vi "Save_File.vi"(6 "Sequence caption in":string, 7 "Path?":bool, 8 "error in (no error)":errorcluster, 9 "Sequence in":string[](array[string]), 10 "Buffer in":string[](array[string]), 11 "Path in":path) -> (0 "error out":errorcluster, 1 "Sequence out":string[](array[string]), 2 "Buffer out":string[](array[string]), 3 "Path out":path, 4 "Sequence caption out":string)   [LabVIEW 2025]
uses:
  <vilib>/Utility/file.llb/Write Delimited Spreadsheet (string).vi
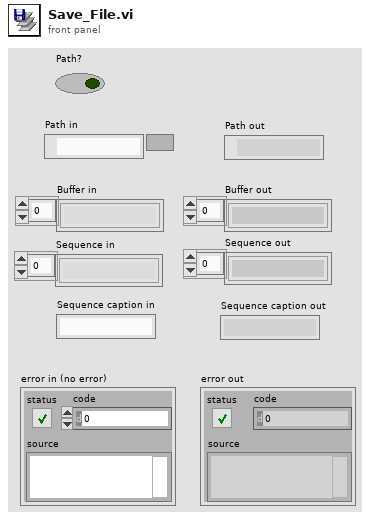
[diagram p1: front panel]
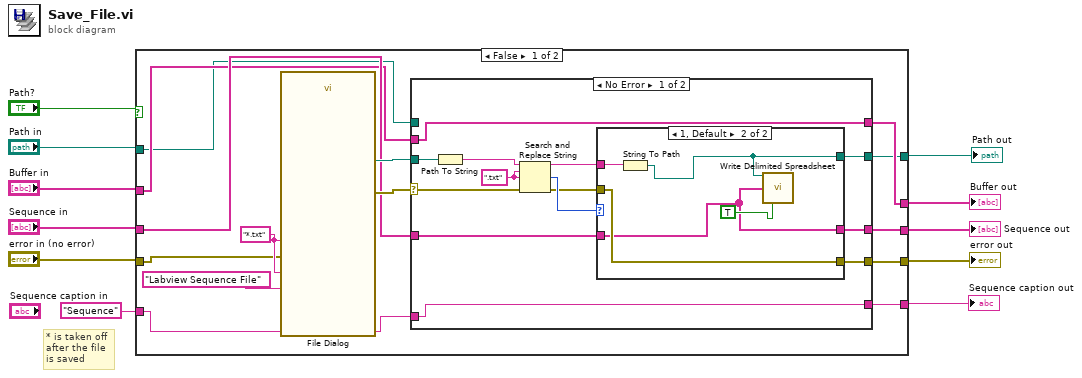
[diagram p0: block diagram]
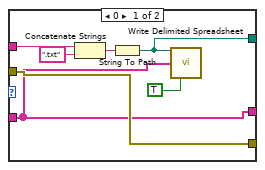
[diagram p2: hidden frame]
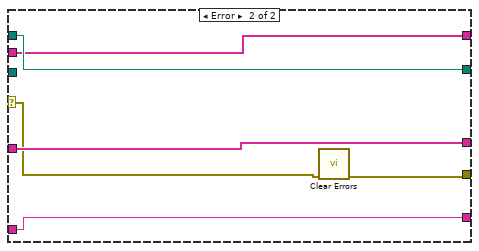
[diagram p3: hidden frame]
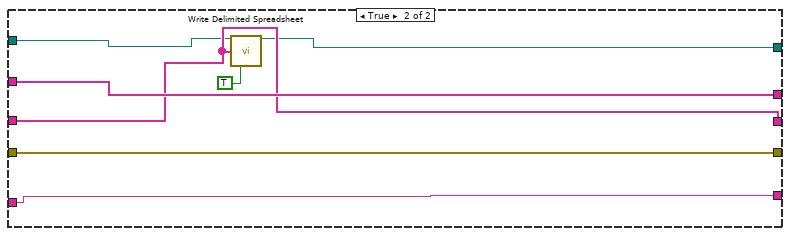
[diagram p4: hidden frame]
diagram:
  # "* is taken off\nafter the file\nis saved"
  n1 = case shown="False" "Path?" {
    tunnel: "Path in" -> [w12 w59]
    tunnel: "Buffer in" -> [w15 w63]
    tunnel: "Sequence in" -> [w18 w60]
    tunnel: "error in (no error)" -> [w21 w62]
    tunnel: [w13 w58] -> w6
    tunnel: [w14 w63] -> w5
    tunnel: [w17 w62] -> w3
    tunnel: [w16 w60] -> w4
    tunnel: "Sequence" ("Sequence caption in") -> [w20 w61]
    tunnel: [w19 w61] -> w2
    frame False {
      w25 = "*.txt" ("default name")
      n2 = call "File Dialog"("default name"=w25, "error in"=w21, "pattern (all files)"=w25, "pattern label"="Labview Sequence File") -> ("selected path"=w23:path, "error out"=w24:errorcluster)  [unwired: 8 in, 2 out]
      n3 = case shown="No Error" w24 {
        selector: w24 -> [w35 w52]
        tunnel: w23 -> [w36 _]
        tunnel: w20 -> [w29 w56]
        tunnel: [w29 w56] -> w19
        tunnel: w18 -> [w32 w55]
        tunnel: [w30 w51] -> w17
        tunnel: [w28 w55] -> w16
        tunnel: w15 -> [w27 w53]
        tunnel: [w27 w53] -> w14
        tunnel: [w26 w54] -> w13
        tunnel: w12 -> [_ w54]
        frame No Error {
          w37 = ".txt" ("search string")
          n4 = Path To String(path=w36) -> (string=w38:string)
          n5 = Search and Replace String(input string=w38, search string=w37, replace string=w37, error in=w35) -> (result string=w33:string, number of replacements=w34:i32, error out=w31:errorcluster)  [unwired: 4 in, 1 out]
          n6 = case shown="1, Default" w34 {
            tunnel: w33 -> [w45 w50]
            tunnel: w32 -> [w40 w46]
            tunnel: w31 -> [w42 w49]
            tunnel: [w42 w49] -> w30
            tunnel: [w40 w46] -> w28
            tunnel: [w39 w48] -> w26
            frame 0 {
              n7 = Concatenate Strings(w45, ".txt" ("string")) -> (w43:string)
              n8 = String To Path(string=w43) -> (path=w39:path)
              n9 = call-poly <vilib>:"Write Delimited Spreadsheet.vi"("file path (dialog if empty)"=w39, "1D data"=w40, "transpose? (no:F)"=TRUE) -> ()  [unwired: 11 in, 2 out]
            }
            frame 1, Default {
              n10 = String To Path(string=w50) -> (path=w48:path)
              n11 = call-poly <vilib>:"Write Delimited Spreadsheet.vi"("file path (dialog if empty)"=w48, "1D data"=w46, "transpose? (no:F)"=TRUE) -> ()  [unwired: 11 in, 2 out]
            }
          }
        }
        frame Error {
          n12 = call <vilib>:"Clear Errors.vi"("error in (no error)"=w52) -> ("error out"=w51:errorcluster)  [unwired: 5 in, 1 out]
        }
      }
    }
    frame True {
      n13 = call-poly <vilib>:"Write Delimited Spreadsheet.vi"("file path (dialog if empty)"=w59, "1D data"=w60, "transpose? (no:F)"=TRUE) -> ("new file path (Not A Path if cancelled)"=w58:path)  [unwired: 11 in, 1 out]
    }
  }
  "Path out" <- w6
  "Buffer out" <- w5
  "Sequence out" <- w4
  "error out" <- w3
  "Sequence caption out" <- w2
